vi "Analyze Event Step 2.vi"(10 "windowed event data":T1) -> (2 "measured data":T3, 3 "measure output.<user name>":T2)   [LabVIEW 2015, in "Engine Simulation Toolkit.lvlib" / "ECU Event Timing.lvlib"]
uses:
  ECU Event Timing.lvlib
  Measured Data.ctl
  Measure Output.ctl
  Windowed Event Data.ctl
  Common/Count Up U8.vi
  Engine Simulation Toolkit.lvlib
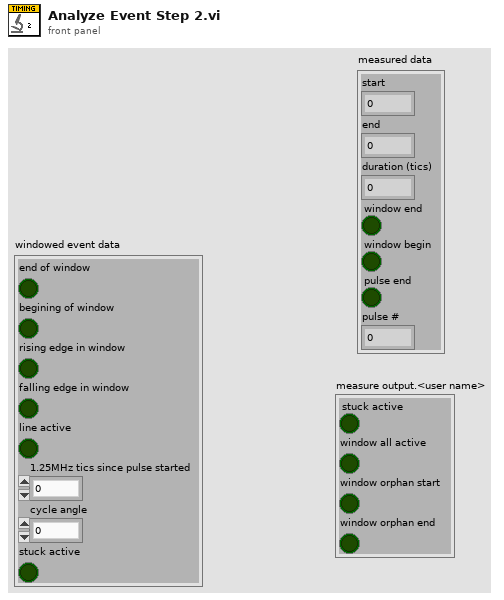
[diagram p1: front panel]
types:
  T1 = typedef "Engine Simulation Toolkit.lvlib/ECU Event Timing.lvlib/Windowed Event Data.ctl" = cluster{"end of window":bool, "begining of window":bool, "rising edge in window":bool, "falling edge in window":bool, "line active":bool, "1.25MHz tics since pulse started":fxp<+,18,18>, "cycle angle":u16, "stuck active":bool}
  T2 = typedef "Engine Simulation Toolkit.lvlib/ECU Event Timing.lvlib/Measure Output.ctl" = cluster{"stuck active":bool, "window all active":bool, "window orphan start":bool, "window orphan end":bool}
  T3 = typedef "Engine Simulation Toolkit.lvlib/ECU Event Timing.lvlib/Measured Data.ctl" = cluster{"start":u16, "end":u16, "duration (tics)":fxp<+,18,18>, "window end":bool, "window begin":bool, "pulse end":bool, "pulse #":u8}
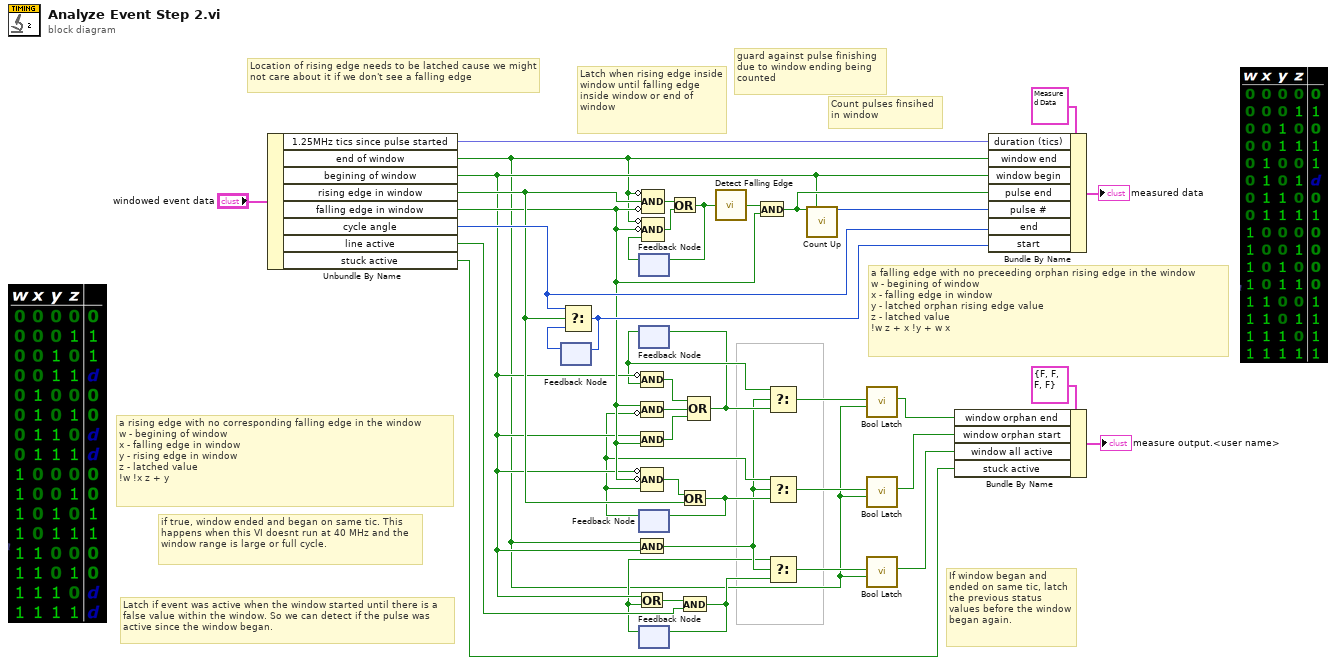
[diagram p0: block diagram]
diagram:
  # "If window began and ended on same tic, latch the previous status values before the window began again."
  # "if true, window ended and began on same tic. This happens when this VI doesnt run at 40 MHz and the window range is large or full cycle."
  # "a falling edge with no preceeding orphan rising edge in the window\nw - begining of window\nx - falling edge in window\ny - latched orphan rising edge value\nz - latched value\n!w z + x !y + w x"
  # "a rising edge with no corresponding falling edge in the window\nw - begining of window\nx - falling edge in window\ny - rising edge in window\nz - latched value\n!w !x z + y"
  # "guard against pulse finishing due to window ending being counted"
  # "Latch if event was active when the window started until there is a false value within the window. So we can detect if the pulse was active since the window began."
  # "Location of rising edge needs to be latched cause we might not care about it if we don't see a falling edge"
  # "Count pulses finsihed  in window"
  # "Latch when rising edge inside window until falling edge inside window or end of window"
  n1 = Unbundle By Name("windowed event data") -> ("1.25MHz tics since pulse started"=w36:fxp<+,18,18>, "end of window"=w2:bool, "begining of window"=w16:bool, "rising edge in window"=w22:bool, "falling edge in window"=w18:bool, "cycle angle"=w38:u16, "line active"=w17:bool, "stuck active"=w15:bool)
  n2 = feedback #1() -> (w39:u16)  [unwired: 1 in]
  n3 = Select(t=w38, s=w22, f=w39) -> (s? t:f=w37:u16)
  n4 = feedback-in #1(w37) -> ()
  n5 = And(x=w16, y=w18) -> (x .and. y?=w20:bool)
  n6 = And(x=w2, y=w16) -> (x .and. y?=w10:bool)
  n7 = feedback #2() -> (w26:bool)  [unwired: 1 in]
  n8 = feedback #3() -> (w12:bool)  [unwired: 1 in]
  n9 = feedback #4() -> (w14:bool)  [unwired: 1 in]
  n10 = feedback #5() -> (w9:bool)  [unwired: 1 in]
  n11 = Or(x=w16, y=w9) -> (x .or. y?=w35:bool)
  n12 = Compound Arithmetic op=AND(invert w16, w12) -> (w21:bool)
  n13 = Compound Arithmetic op=AND(w18, invert w14) -> (w19:bool)
  n14 = Compound Arithmetic op=AND(invert w16, invert w18, w14) -> (w23:bool)
  n15 = Compound Arithmetic op=AND(invert w2, w22, invert w18) -> (w28:bool)
  n16 = Compound Arithmetic op=AND(invert w2, invert w18, w26) -> (w27:bool)
  n17 = Or(x=w28, y=w27) -> (x .or. y?=w29:bool)
  n18 = feedback-in #2(w29) -> ()
  n19 = Or(x=w23, y=w22) -> (x .or. y?=w13:bool)
  n20 = feedback-in #4(w13) -> ()
  n21 = And(x=w35, y=w17) -> (x .and. y?=w8:bool)
  n22 = feedback-in #5(w8) -> ()
  n23 = Compound Arithmetic op=OR(w21, w19, w20) -> (w11:bool)
  n24 = feedback-in #3(w11) -> ()
  n25 = call "Detect Falling Edge.vi"("signal"=w29) -> ("edge detected"=w24:bool)  [unwired: 14 in]
  n26 = And(x=w24, y=w18) -> (x .and. y?=w25:bool)
  n27 = Select(t=w12, s=w10, f=w11) -> (s? t:f=w7:bool)
  n28 = Select(t=w14, s=w10, f=w13) -> (s? t:f=w5:bool)
  n29 = Select(t=w9, s=w10, f=w8) -> (s? t:f=w3:bool)
  n30 = call-poly "Count Up.vi"("increment"=w25, "reset"=w16) -> ("count out"=w40:u8)  [unwired: 13 in]
  n31 = call "Bool Latch.vi"("set"=w2, "value"=w7) -> ("out"=w6:bool)  [unwired: 9 in]
  n32 = call "Bool Latch.vi"("set"=w2, "value"=w5) -> ("out"=w4:bool)  [unwired: 9 in]
  n33 = call "Bool Latch.vi"("set"=w2, "value"=w3) -> ("out"=w1:bool)  [unwired: 9 in]
  n34 = Bundle By Name(cluster=T2 {"stuck active"=FALSE, "window all active"=FALSE, "window orphan start"=FALSE, "window orphan end"=FALSE} ("output"), "window orphan end"=w6, "window orphan start"=w4, "window all active"=w1, "stuck active"=w15) -> (→"measure output.<user name>":T2)
  n35 = Bundle By Name(cluster=T3 {"start"=0, "end"=0, "duration (tics)"=0.0, "window end"=FALSE, "window begin"=FALSE, "pulse end"=FALSE, "pulse #"=0} ("output"), "duration (tics)"=w36, "window end"=w2, "window begin"=w16, "pulse end"=w25, "pulse #"=w40, "end"=w38, "start"=w37) -> (→"measured data":T3)
